vi "Mail weather report at last.vi"() -> (3 "Array 3":T1(array[cluster]))   [LabVIEW 2013]
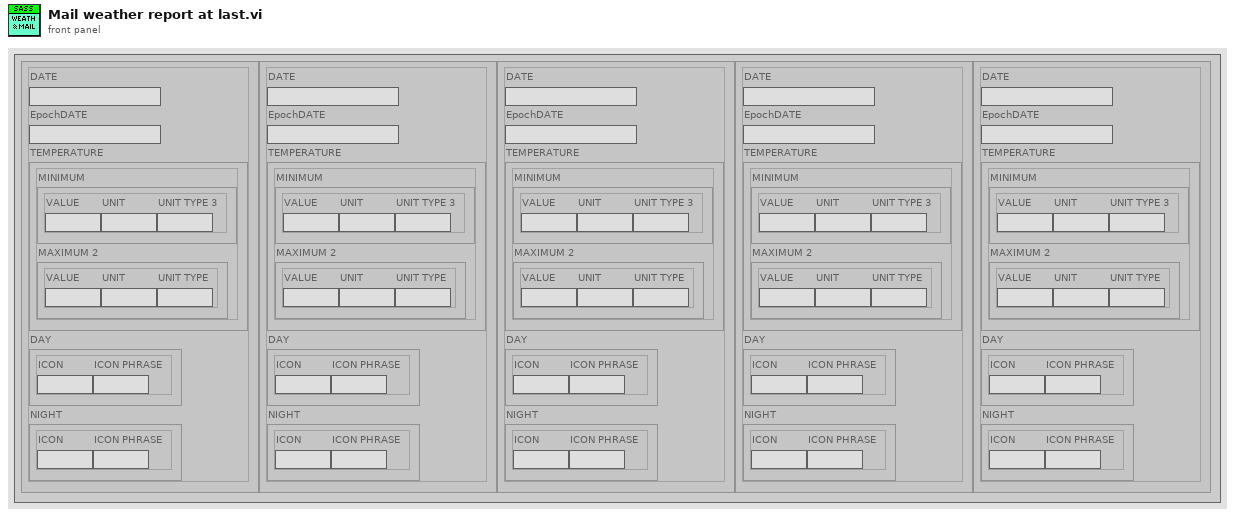
[diagram p1: front panel]
types:
  T1 = cluster{"DATE":string, "EpochDATE":string, "TEMPERATURE":cluster{"MINIMUM":cluster{"VALUE":string, "UNIT":string, "UNIT TYPE 3":string}, "MAXIMUM 2":cluster{"VALUE":string, "UNIT":string, "UNIT TYPE":string}}, "DAY ":cluster{"ICON":string, "ICON PHRASE":string}, "NIGHT":cluster{"ICON":string, "ICON PHRASE":string}}[]
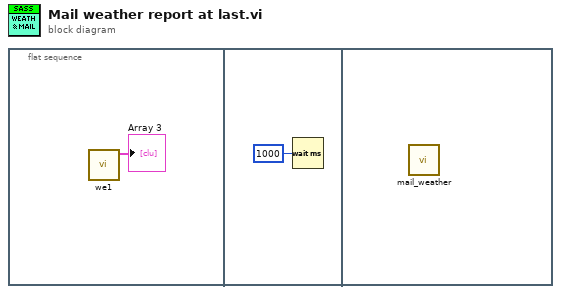
[diagram p0: block diagram]
diagram:
  n1 = flat-sequence {
    frame #0 {
      n2 = call "we1.vi"() -> ("Array 3"=→"Array 3":T1)  [unwired: 11 in]
    }
    frame #1 {
      n3 = Wait (ms)(milliseconds to wait=u32 1000) -> ()  [unwired: 1 out]
    }
    frame #2 {
      n4 = call "mail_weather.vi"() -> ()  [unwired: 12 in]
    }
  }
